vi "Relation.vi"(11 "Base Sender in":refnum<class "Base Sender.lvclass">) -> (2 "Relation":T1)   [LabVIEW 2020, in "jettl.lvlib" / "Sender.lvlib" / "Base Sender.lvclass"]
uses:
  Base Sender.lvclass
  Relation.ctl
  Base Sender.lvclass/Base Sender.ctl
  Sender.lvlib
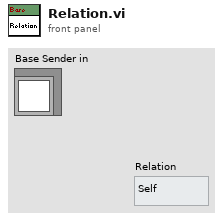
[diagram p1: front panel]
types:
  T1 = typedef "jettl.lvlib/Sender.lvlib/Relation.ctl" = enum16{"Self", "Creator", "Created"}
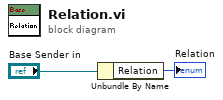
[diagram p0: block diagram]
diagram:
  n1 = Unbundle By Name("Base Sender in") -> ("Relation"=→"Relation":T1)
